vi "Cleanup.vi"(8 "error in (no error)":errorcluster, 11 "Symbol Map in":refnum<class "Symbol Map.lvclass">) -> (0 "error out":errorcluster)   [LabVIEW 2020, in "PicoG-ParserLexer.lvlib" / "Symbol Map.lvclass"]
uses:
  Symbol Map.lvclass
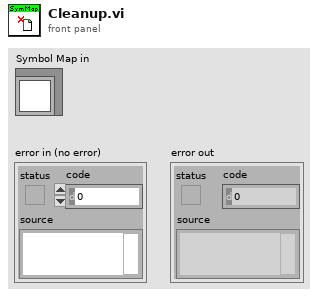
[diagram p1: front panel]
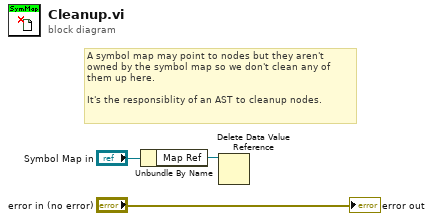
[diagram p0: block diagram]
diagram:
  # "A symbol map may point to nodes but they aren't owned by the symbol map so we don't clean any of them up here.\n\nIt's the responsiblity of an AST to cleanup nodes."
  n1 = Unbundle By Name("Symbol Map in") -> ("Map Ref"=w1:refnum<data-value>)
  n2 = Delete Data Value Reference(data value reference=w1) -> ()  [unwired: 1 in, 2 out]
  "error out" <- "error in (no error)"
